vi "DFD Chebyshev Order Estimation.vi"(6 "fs [Hz]":dbl=1.0 format="%.2f", 7 "filter type":T3(ring), 8 "error in (no error)":errorcluster, 10 "ripple specs":T1={"passband"=0.1, "stopband"=60.0, "dB/linear? (T: dB)"=TRUE}, 11 "freq specs [Hz]":T2={"fpass 1"=0.2, "fstop 1"=0.3, "fpass 2 "=0.0, "fstop 2"=0.0}) -> (0 "error out":errorcluster, 1 "low cutoff freq [Hz]":dbl, 2 "high cutoff freq [Hz]":dbl, 3 "estimated order":i32, 4 "passband ripple [dB]":dbl format="%.2f")   [LabVIEW 2017, in "NI_DigFilterLicensed.lvlib"]
doc: "Estimates the Chebyshev I filter order."
uses:
  <vilib>/addons/Digital Filter Design/NI_DigFilterLicensed.lvlib
  <vilib>/addons/Digital Filter Design/_Objects.llb/DFD Filter Frequence Specification (Design).ctl
  <vilib>/addons/Digital Filter Design/_Objects.llb/DFD Filter Ripple Specification (Design).ctl
  <vilib>/addons/Digital Filter Design/NI_DigFilter_Design.lvlib
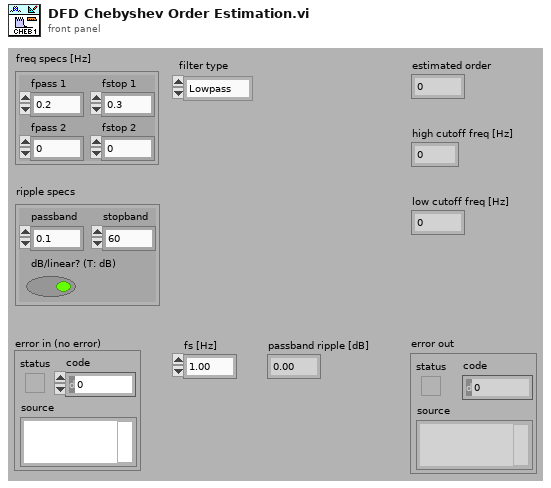
[diagram p1: front panel]
types:
  T1 = typedef "NI_DigFilterLicensed.lvlib/DFD Filter Ripple Specification (Design).ctl" = cluster{"passband":dbl, "stopband":dbl, "dB/linear? (T: dB)":bool}
  T2 = typedef "NI_DigFilterLicensed.lvlib/DFD Filter Frequence Specification (Design).ctl" = cluster{"fpass 1":dbl, "fstop 1":dbl, "fpass 2 ":dbl, "fstop 2":dbl}
  T3 = enum16{"Lowpass", "Highpass", "Bandpass", "Bandstop"}
  T4 = enum16{"Butterworth", "Chebyshev", "Inverse Chebyshev", "Elliptic", "Bessel"}
  T5 = cluster{"passband ripple":dbl, "stopband atten":dbl}
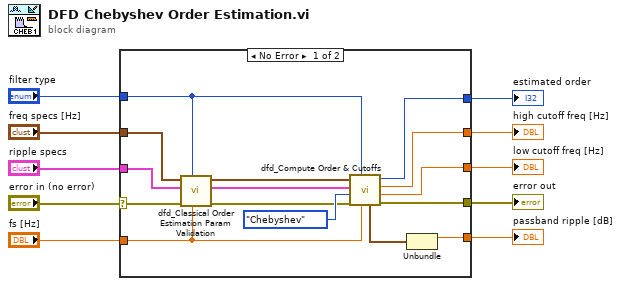
[diagram p0: block diagram]
diagram:
  n1 = case shown="No Error" "error in (no error)" {
    selector: "error in (no error)" -> [w11 w26]
    tunnel: "fs [Hz]" -> [w25 _]
    tunnel: "filter type" -> [w24 _]
    tunnel: "freq specs [Hz]" -> [w23 _]
    tunnel: "ripple specs" -> [w22 _]
    tunnel: [w20 _] -> w6
    tunnel: [w18 w26] -> w5
    tunnel: [w14 _] -> w4
    tunnel: [w13 _] -> w3
    tunnel: [w12 _] -> w2
    frame No Error {
      n2 = call <vilib>:"dfd_Classical Order Estimation Param Validation.vi"("fs [Hz]"=w25, "filter type"=w24, "error in (no error)"=w11, "ripple specs"=w22, "freq specs [Hz]"=w23) -> ("error out"=w19:errorcluster, "dup ripple specs"=w16:T1, "dup freq specs [Hz]"=w17:T2)  [unwired: 1 in, 3 out]
      n3 = call <vilib>:"dfd_Compute Order & Cutoffs.vi"("fs [Hz]"=w25, "filter type"=w24, "error in (no error)"=w19, "design method"=T4."Chebyshev", "ripple specs"=w16, "freq specs [Hz]"=w17) -> ("error out"=w18:errorcluster, "low cutoff freq: fl"=w14:dbl, "high cutoff freq: fh"=w13:dbl, "N"=w12:i32, "ripples [dB]"=w15:T5)  [unwired: 1 out]
      n4 = Unbundle(w15) -> ("passband ripple"=w20:dbl)  [unwired: 1 out]
    }
    frame Error {
    }
  }
  "estimated order" <- w2
  "error out" <- w5
  "passband ripple [dB]" <- w6
  "high cutoff freq [Hz]" <- w3
  "low cutoff freq [Hz]" <- w4
